vi "Instrument_Setting.vi"(8 "错误输入（无错误）":errorcluster, 9 "id":string[](array[string]), 10 "Get_USB_Resouce":string[](array[string]), 11 "Address Cluster":T2={"SPU"=refnum, "MPM"=[], "Port_Count"=0.0, "MPM_Count"=0.0, "SPU_Resource"=[], "USB_Resource"=[], "MPM_Communicater"="", "MPM_Count"=0.0, "MPM_Address"=[], "MPM_Portnumber"=[], "SPU_DeviveID"="", "MPM_communcation_method"=[], "TSL_sweepstartwave"=0.0, "TSL_sweepstopwave"=0.0, "TSL_Address"="", "TSL_Communicater"="", "TSL"=refnum, "tsl_communcation_method"=3, "TSL_Portnumber"=0.0, "PCU"=refnum, "PCU_Communicater"="", "PCU_Address"="", "PCU_Portnumber"=0.0, "PCU_useing_internal_DAQ"=FALSE, "PCU_communcation_method"=0} {"PCU_communcation_method" items=["GPIB", "C232C", "TCPIP", "USB"]; "tsl_communcation_method" items=["GPIB", "C232C", "TCPIP", "USB"]; "MPM_communcation_method" items=["GPIB", "C232C", "TCPIP", "USB"]}) -> (0 "错误输出":errorcluster, 2 "PowerMonitorType":enum16{"DAQ", "MPM_220", "TSL_LOGG"}(ring), 3 "Address Cluster out":T2={"SPU"=refnum, "MPM"=[], "Port_Count"=0.0, "MPM_Count"=0.0, "SPU_Resource"=[], "USB_Resource"=[], "MPM_Communicater"="", "MPM_Count"=0.0, "MPM_Address"=[], "MPM_Portnumber"=[], "SPU_DeviveID"="", "MPM_communcation_method"=[], "TSL_sweepstartwave"=0.0, "TSL_sweepstopwave"=0.0, "TSL_Address"="", "TSL_Communicater"="", "TSL"=refnum, "tsl_communcation_method"=3, "TSL_Portnumber"=0.0, "PCU"=refnum, "PCU_Communicater"="", "PCU_Address"="", "PCU_Portnumber"=0.0, "PCU_useing_internal_DAQ"=FALSE, "PCU_communcation_method"=0} {"PCU_communcation_method" items=["GPIB", "C232C", "TCPIP", "USB"]; "tsl_communcation_method" items=["GPIB", "C232C", "TCPIP", "USB"]; "MPM_communcation_method" items=["GPIB", "C232C", "TCPIP", "USB"]})   [LabVIEW 2017]
doc: "Setting Form"
uses:
  CTL/Address Cluster.ctl
  D:/test/PDLSTS/LV_PDL LvVer17.0/LV_PDL_x64/DLL/InstrumentDLL.dll
  DLL/InstrumentDLL.dll
  Share/Product_PCU.vi
  Share/MPM_PowerMonitorType.vi
panel:
  out "Enable220Flag":bool
  in  "Preformence":enum32{"High-Spec", "Standard"}(radio) caption="Preformance"
  in  "Product_MPM":enum32{"MPM-210/210H", "MPM-220"}(radio) caption="Product"
  in  "txtpcu_ipadd":string caption="IP Address"
  in  "txtpcu_lanport":i32=5000 caption="LAN Port"
  in  "txtpcu_gpibadd":i32=1 caption="GPIB Address"
  in  "cmbpcu_usbresource":u16(ring) caption="Usb resouce"
  in  "Communication_PCU":T1(radio) caption="Communication"
  in  "Product_PCU":enum32{"rdopcu100", "rdopcu110"}(radio) caption="Product"
  out "Boolean":bool=TRUE
  in  "Port_Count":i32
  in  "btnconnect":bool
  in  "cmbSPU_dev":u16(ring) caption="SPU" items=["Dev3"]
  in  "IP Address_MPM 2":string caption="IP Address"
  in  "LAN Port_MPM 2":dbl caption="LAN Port"
  in  "GPIB Address_MPM 2":i32 caption="GPIB Address"
  in  "chkmulti_dev":bool
  in  "IP Address_MPM":string caption="IP Address"
  in  "LAN Port_MPM":dbl=5000.0 caption="LAN Port"
  in  "GPIB Address_MPM":i32=14 caption="GPIB Address"
  in  "Communication_MPM":enum32{"rdiGPIB_MPM", "rdiLAN_MPM"}(radio) caption="Communication"
  in  "IP Address_TSL1":string caption="IP Address"
  in  "LAN Port_TSL1":i32 caption="LAN Port"
  in  "GPIB Address_TSL1":i32=1 caption="GPIB Address"
  in  "Usb resouce_TSL1":u16(ring) caption="Usb resouce"
  in  "Communication_TSL":T3(radio) caption="Communication"
  in  "Product_TSL":enum32{"rdo550_TSL", "rdo570_TSL"}(radio) caption="Product"
  # "TSL"
  # "MPM"
  # "Device2"
  # "Device1"
  # "PCU"
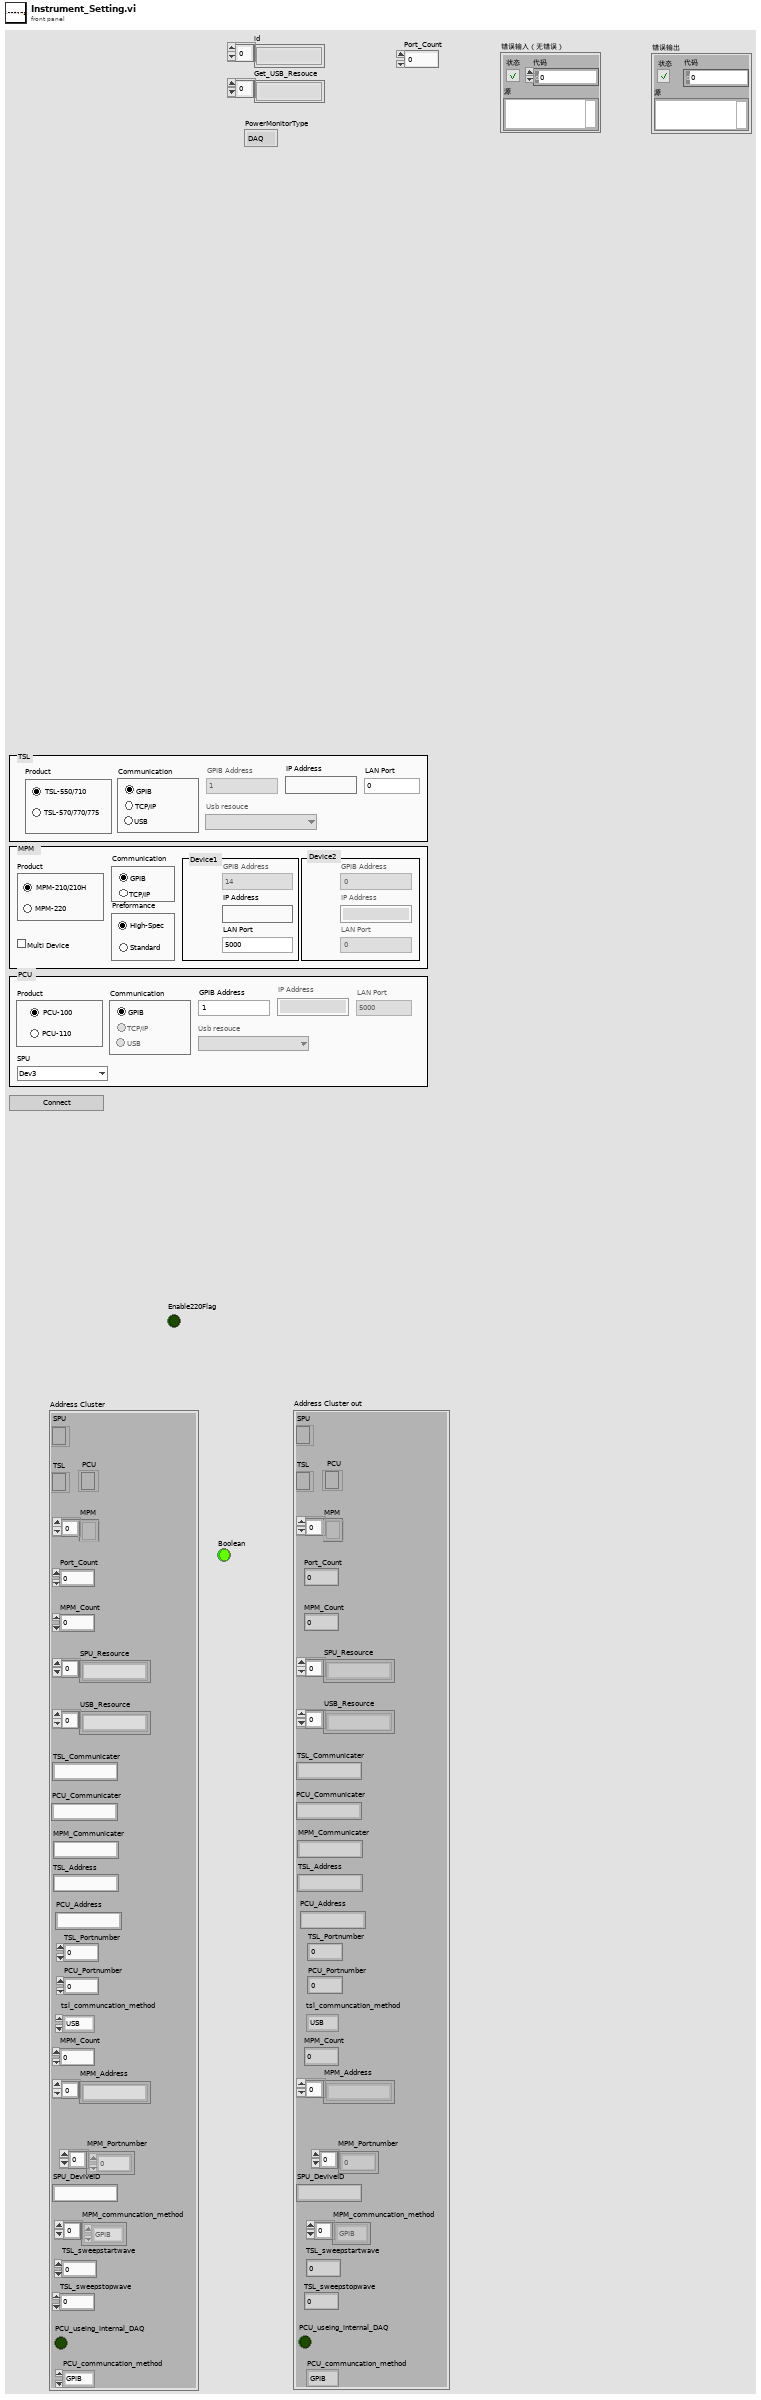
[diagram p1: front panel]
types:
  T1 = enum32{"rdopcu_gpib", "rdopcu_lan", "rdopcu_usb"}
  T2 = typedef "Address Cluster.ctl" = cluster{"SPU":refnum<k24>, "MPM":refnum<k24>[], "Port_Count":dbl, "MPM_Count":dbl, "SPU_Resource":string[], "USB_Resource":string[], "MPM_Communicater":string, "MPM_Count":dbl, "MPM_Address":string[], "MPM_Portnumber":dbl[], "SPU_DeviveID":string, "MPM_communcation_method":i32[], "TSL_sweepstartwave":dbl, "TSL_sweepstopwave":dbl, "TSL_Address":string, "TSL_Communicater":string, "TSL":refnum<k24>, "tsl_communcation_method":i32, "TSL_Portnumber":dbl, "PCU":refnum<k24>, "PCU_Communicater":string, "PCU_Address":string, "PCU_Portnumber":dbl, "PCU_useing_internal_DAQ":bool, "PCU_communcation_method":i32}
  T3 = enum32{"rdiGPIB_TSL", "rdiLAN_TSL", "rdiUSB_TSL"}
  T4 = enum8{"Enabled", "Disabled", "Disabled and Grayed Out"}
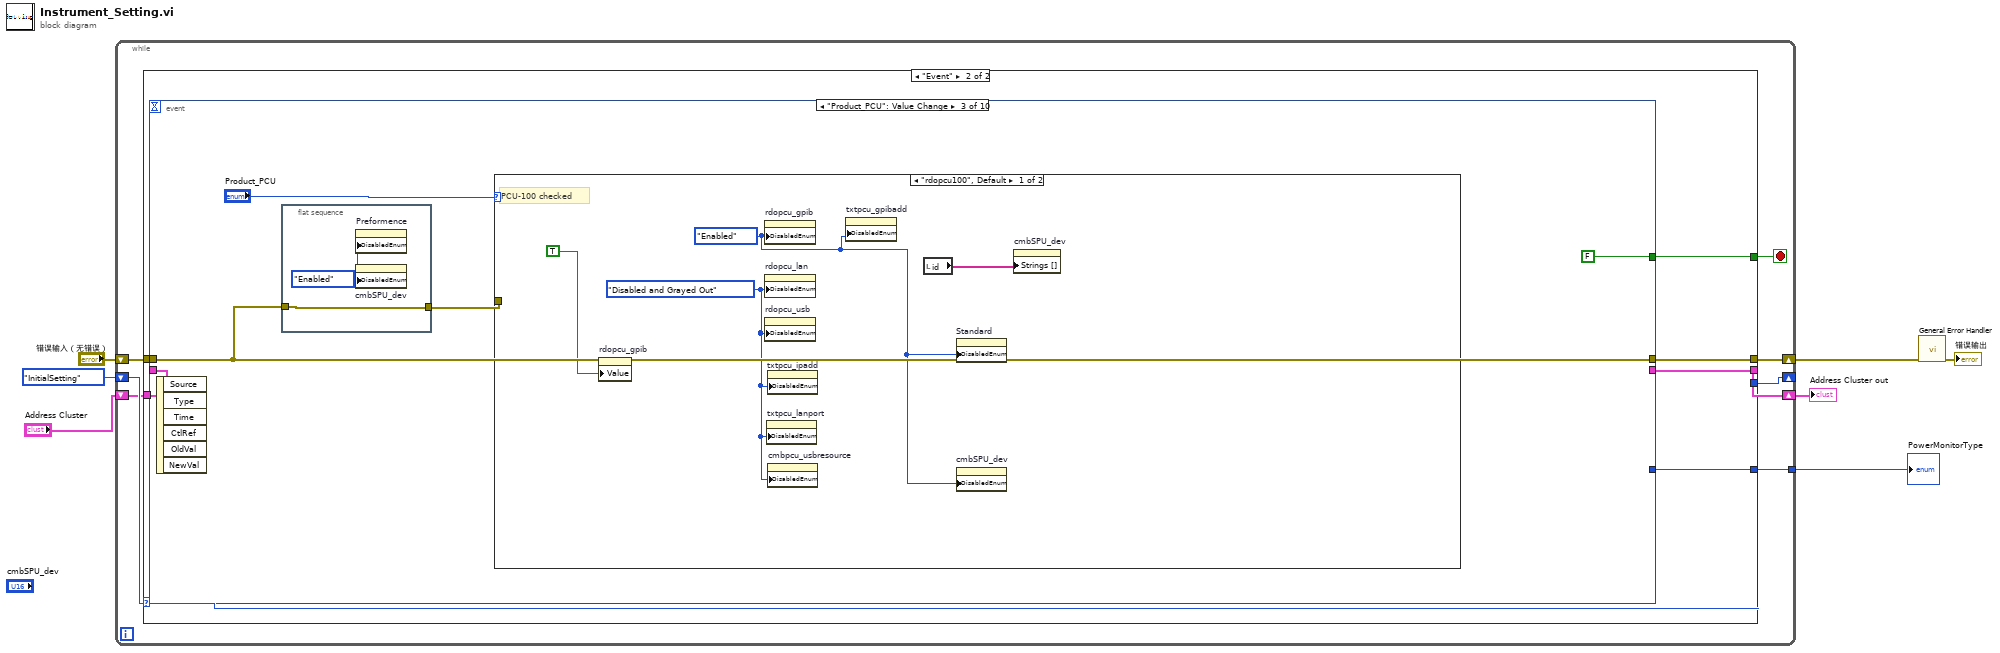
[diagram p0: block diagram]
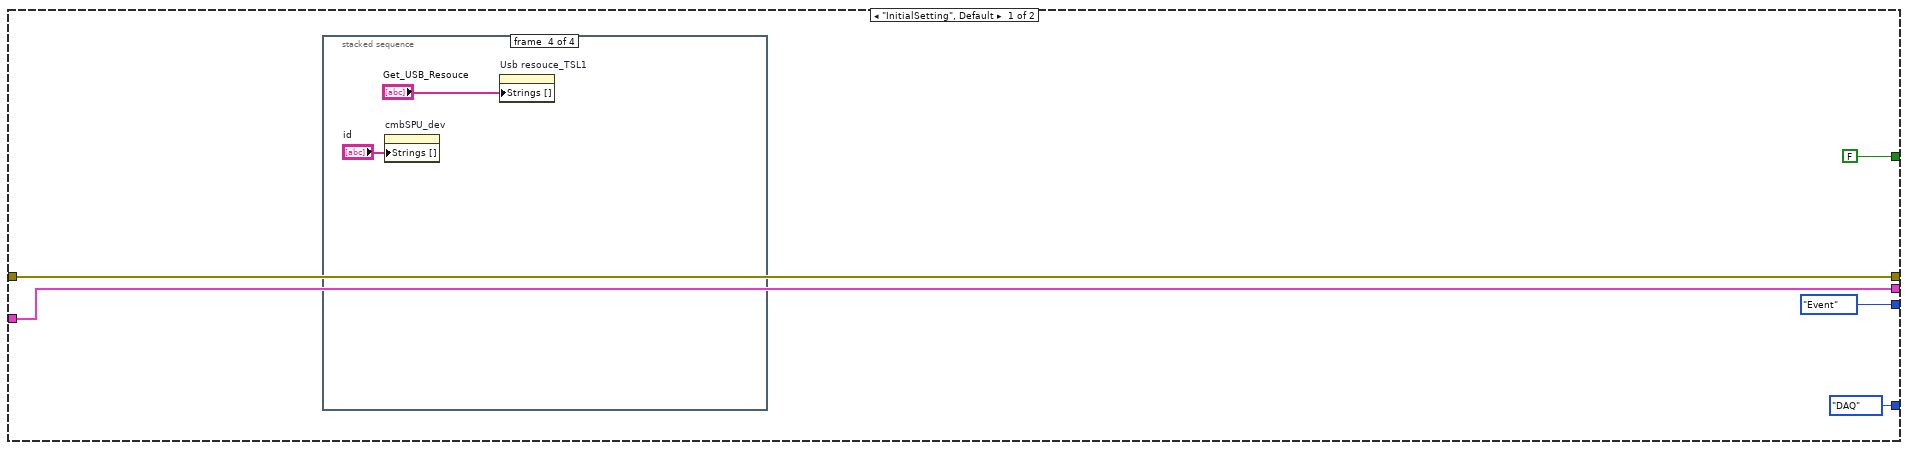
[diagram p2: hidden frame]
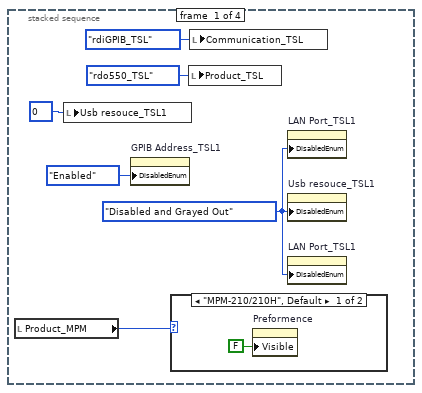
[diagram p3: hidden frame]
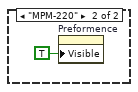
[diagram p4: hidden frame]
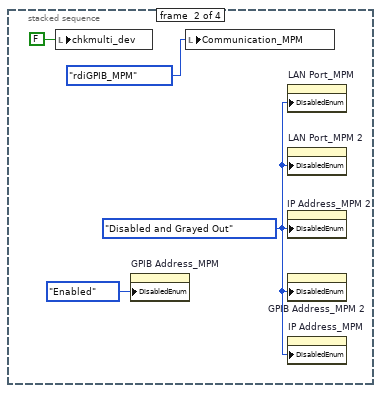
[diagram p5: hidden frame]
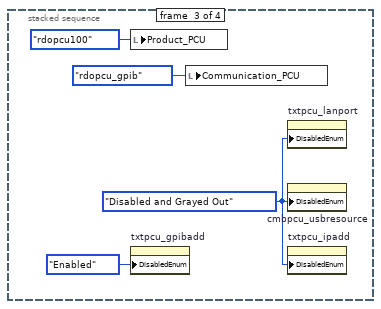
[diagram p6: hidden frame]
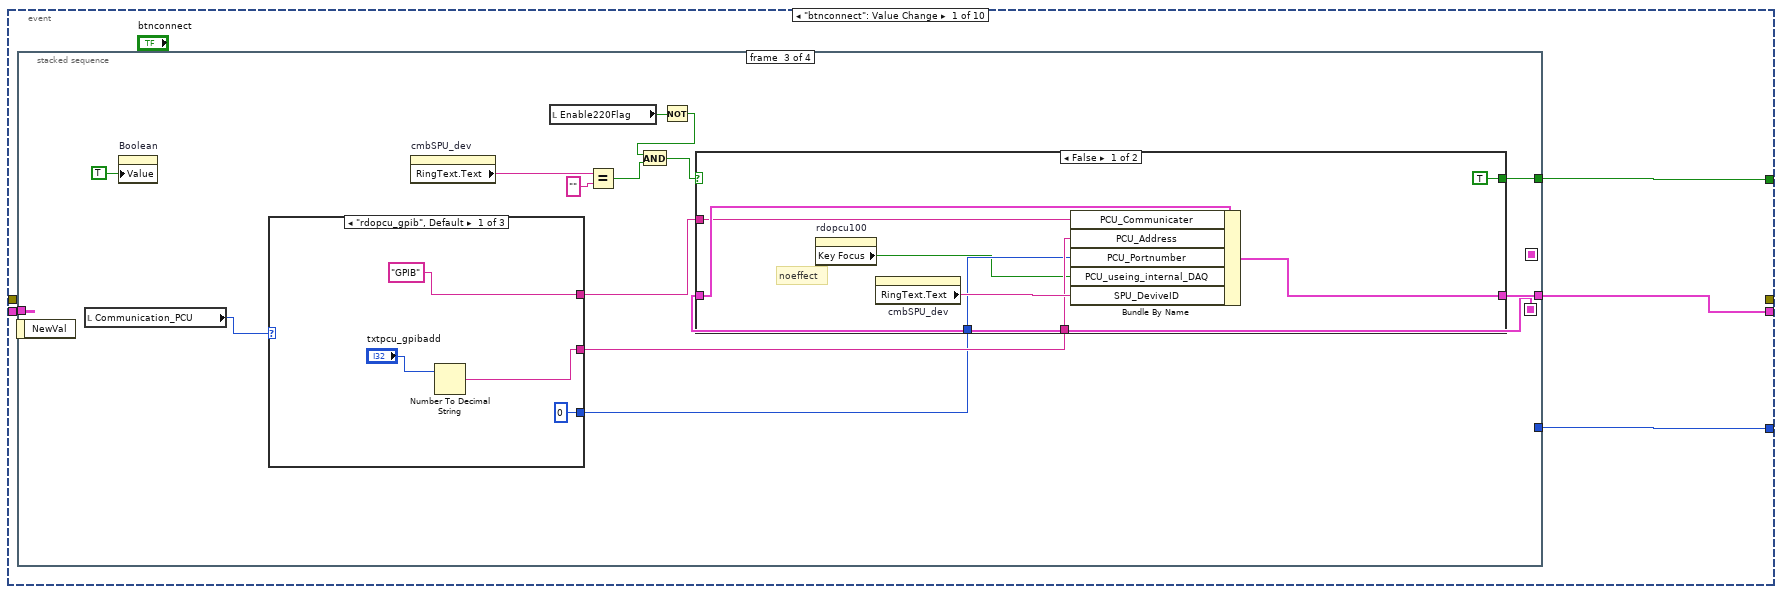
[diagram p7: hidden frame]
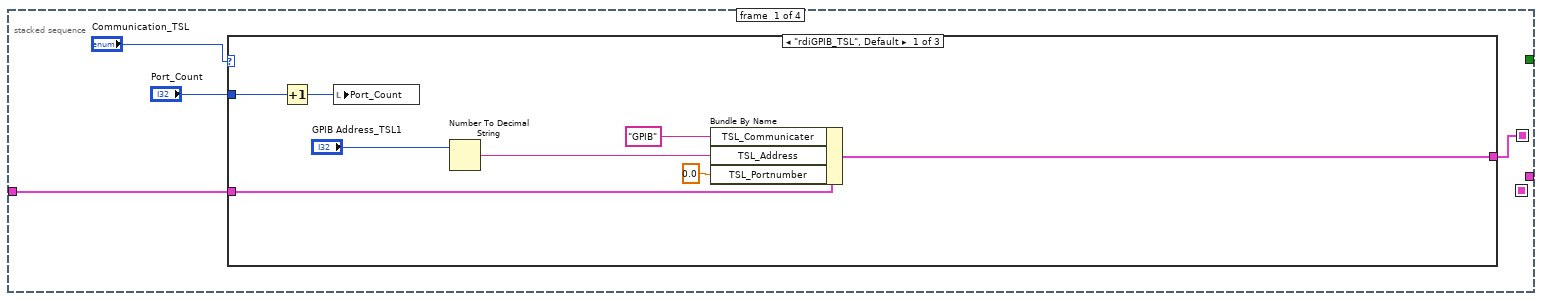
[diagram p8: hidden frame]
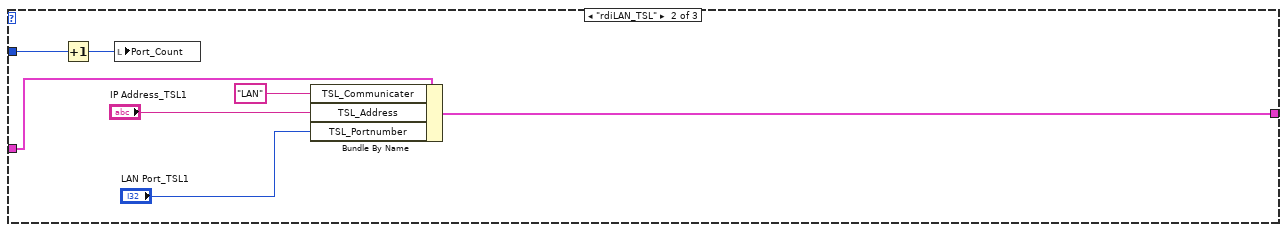
[diagram p9: hidden frame]
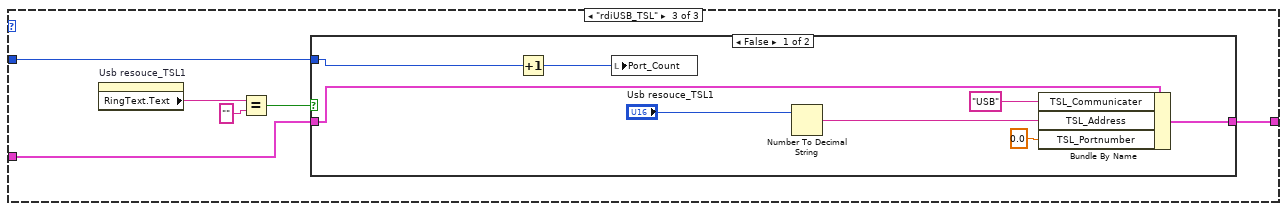
[diagram p10: hidden frame]
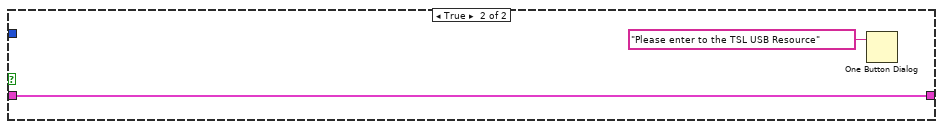
[diagram p11: hidden frame]
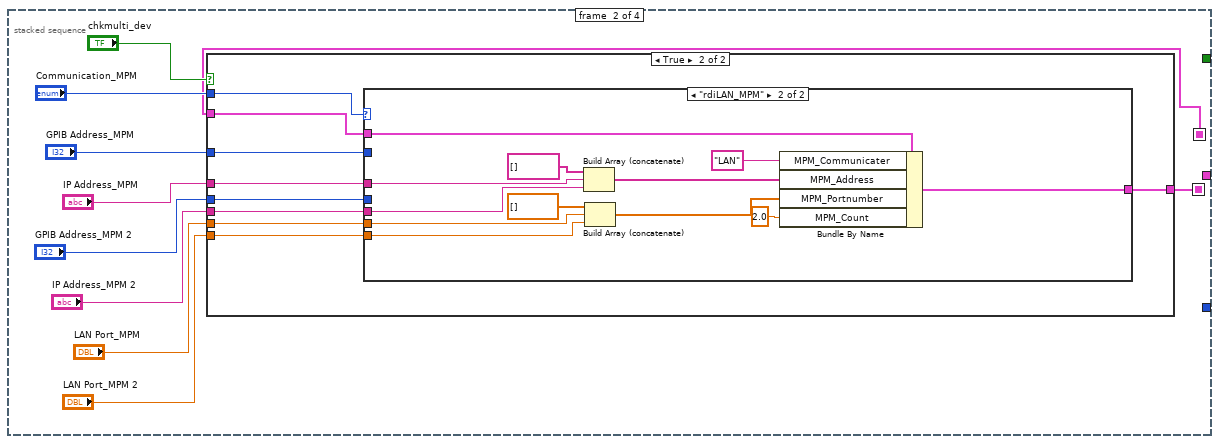
[diagram p12: hidden frame]
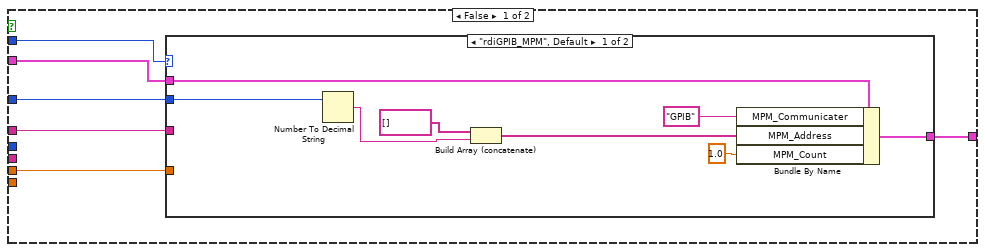
[diagram p13: hidden frame]
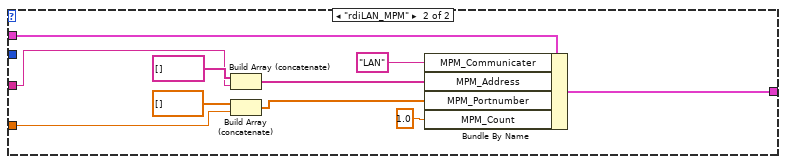
[diagram p14: hidden frame]
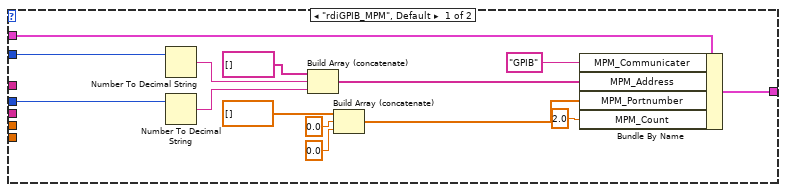
[diagram p15: hidden frame]
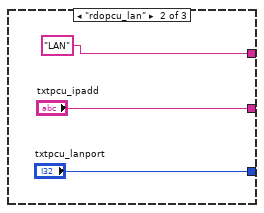
[diagram p16: hidden frame]
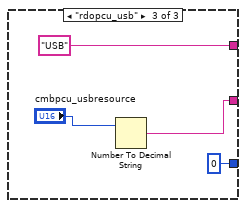
[diagram p17: hidden frame]
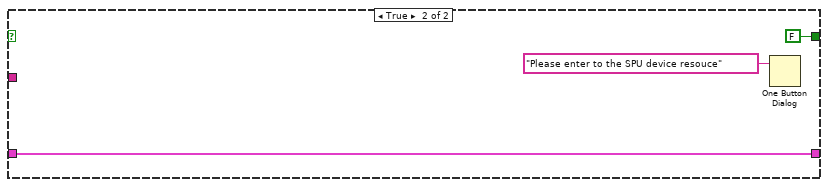
[diagram p18: hidden frame]
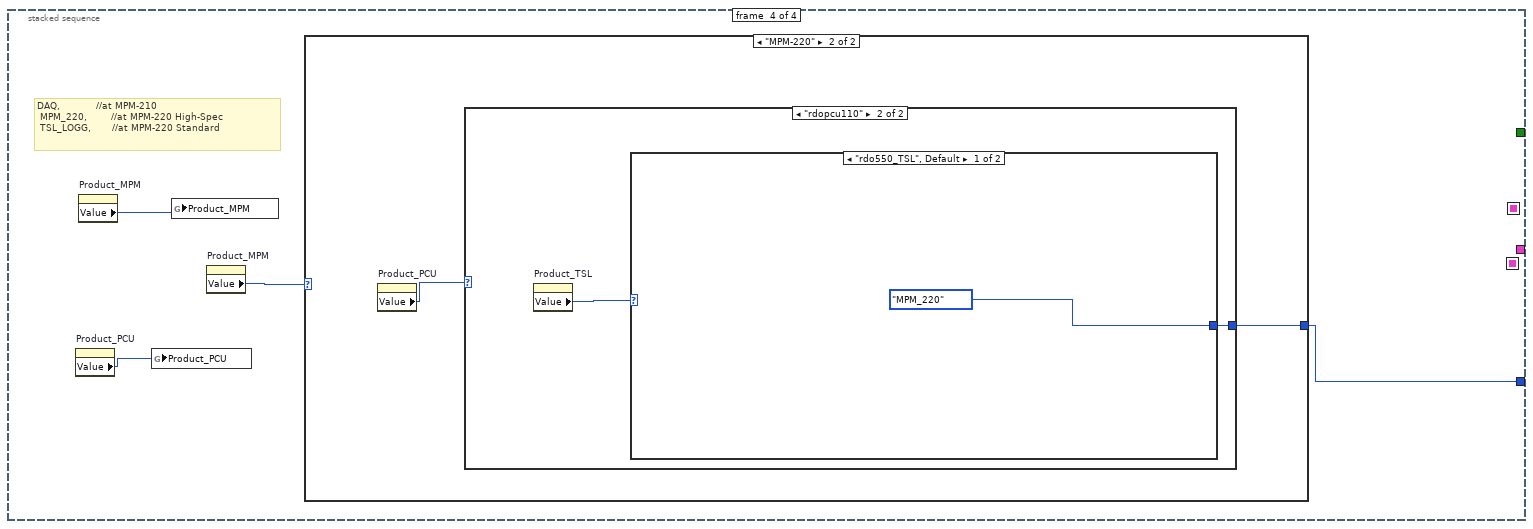
[diagram p19: hidden frame]
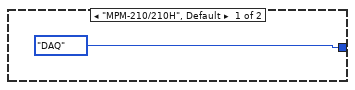
[diagram p20: hidden frame]
diagram:
  n1 = while {
    shift-right: [w14] -> w5
    shift-left: "错误输入（无错误）" -> [w15]
    shift-right: [w12] -> _
    shift-left: enum16{"InitialSetting", "Event", "Set", "Exit"}."InitialSetting" -> [w13]
    shift-right: [w10] -> w2
    shift-left: "Address Cluster" -> [w11]
    tunnel: [w8] -> w1
    stop <- w9 stop-if-true
    n2 = case shown="\"Event\"" w13 {
      selector: w13 -> [_ w41]
      tunnel: w15 -> [w17 w45]
      tunnel: [w17 w44] -> w14
      tunnel: [FALSE ("status") w40] -> w9
      tunnel: [enum16{"InitialSetting", "Event", "Set", "Exit"}."Event" w41] -> w12
      tunnel: w11 -> [w18 w43]
      tunnel: [w18 w42] -> w10
      tunnel: [enum16{"DAQ", "MPM_220", "TSL_LOGG"}."DAQ" ("f") w39] -> w8
      frame "InitialSetting", Default {
        n3 = stacked-sequence {
          frame #0 {
            w25 = T4."Disabled and Grayed Out" ("禁用")
            w26 = u16 0 items=[""] ("Usb resouce_TSL1")
            n4 = local read "Product_MPM"() -> (w21:enum32{"MPM-210/210H", "MPM-220"})
            n5 = local write "Usb resouce_TSL1"(w26) -> ()
            n6 = property on="GPIB Address_TSL1" class="DigNum (strict)"("DisabledEnum"=T4."Enabled" ("禁用")) -> ()  [unwired: 2 in, 2 out]
            n7 = case shown="\"MPM-210/210H\", Default" w21 {
              frame "MPM-210/210H", Default {
                n8 = property on="Preformence" class="RadioBtnsControl (strict)"("Visible"=FALSE) -> ()  [unwired: 2 in, 2 out]
              }
              frame "MPM-220" {
                n9 = property on="Preformence" class="RadioBtnsControl (strict)"("Visible"=TRUE) -> ()  [unwired: 2 in, 2 out]
              }
            }
            n10 = local write "Product_TSL"(enum32{"rdo550_TSL", "rdo570_TSL"}."rdo550_TSL" ("Product_TSL")) -> ()
            n11 = local write "Communication_TSL"(T3."rdiGPIB_TSL" ("Communication_TSL")) -> ()
            n12 = property on="LAN Port_TSL1" class="DigNum (strict)"("DisabledEnum"=w25) -> ()  [unwired: 2 in, 2 out]
            n13 = property on="Usb resouce_TSL1" class="Ring (strict)"("DisabledEnum"=w25) -> ()  [unwired: 2 in, 2 out]
            n14 = property on="LAN Port_TSL1" class="DigNum (strict)"("DisabledEnum"=w25) -> ()  [unwired: 2 in, 2 out]
          }
          frame #1 {
            w29 = T4."Disabled and Grayed Out" ("禁用")
            n15 = local write "chkmulti_dev"(FALSE ("chkmulti_dev")) -> ()
            n16 = property on="GPIB Address_MPM" class="DigNum (strict)"("DisabledEnum"=T4."Enabled" ("禁用")) -> ()  [unwired: 2 in, 2 out]
            n17 = local write "Communication_MPM"(enum32{"rdiGPIB_MPM", "rdiLAN_MPM"}."rdiGPIB_MPM" ("Communication_MPM")) -> ()
            n18 = property on="LAN Port_MPM" class="DigNum (strict)"("DisabledEnum"=w29) -> ()  [unwired: 2 in, 2 out]
            n19 = property on="LAN Port_MPM 2" class="DigNum (strict)"("DisabledEnum"=w29) -> ()  [unwired: 2 in, 2 out]
            n20 = property on="IP Address_MPM 2" class="Str"("DisabledEnum"=w29) -> ()  [unwired: 2 in, 2 out]
            n21 = property on="GPIB Address_MPM 2" class="DigNum (strict)"("DisabledEnum"=w29) -> ()  [unwired: 2 in, 2 out]
            n22 = property on="IP Address_MPM" class="Str"("DisabledEnum"=w29) -> ()  [unwired: 2 in, 2 out]
          }
          frame #2 {
            w33 = T4."Disabled and Grayed Out" ("禁用")
            n23 = local write "Product_PCU"(enum32{"rdopcu100", "rdopcu110"}."rdopcu100" ("Product_PCU")) -> ()
            n24 = property on="txtpcu_gpibadd" class="DigNum (strict)"("DisabledEnum"=T4."Enabled" ("禁用")) -> ()  [unwired: 2 in, 2 out]
            n25 = local write "Communication_PCU"(T1."rdopcu_gpib" ("Communication_PCU")) -> ()
            n26 = property on="txtpcu_lanport" class="DigNum (strict)"("DisabledEnum"=w33) -> ()  [unwired: 2 in, 2 out]
            n27 = property on="cmbpcu_usbresource" class="Ring (strict)"("DisabledEnum"=w33) -> ()  [unwired: 2 in, 2 out]
            n28 = property on="txtpcu_ipadd" class="Str"("DisabledEnum"=w33) -> ()  [unwired: 2 in, 2 out]
          }
          frame #3 {
            n29 = property on="cmbSPU_dev" class="Ring (strict)"("Strings []"="id") -> ()  [unwired: 2 in, 2 out]
            n30 = property on="Usb resouce_TSL1" class="Ring (strict)"("Strings []"="Get_USB_Resouce") -> ()  [unwired: 2 in, 2 out]
          }
        }
      }
      frame "Event" {
        n31 = event shown="[2] \"Product_PCU\": Value Change" {
          selector: _ -> [_ _ _ _ _ _ _ _ _ _]
          dyn-events: _ -> [_ _ _ _ _ _ _ _ _ _]
          timeout: _ -> [_ _ _ _ _ _ _ _ _ _]
          tunnel: w45 -> [_ w212 w231 w256 w273 w274 _ w290 w299 _]
          tunnel: [_ w212 w231 w256 w273 w274 _ w290 w299 _] -> w44
          tunnel: w43 -> [w49 _ _ _ _ _ _ _ _ w314]
          tunnel: [w48 _ _ _ _ _ _ _ _ w314] -> w42
          tunnel: [w47 FALSE ("y") FALSE ("y") _ _ FALSE ("y") _ FALSE ("y") FALSE ("y") TRUE ("y")] -> w40
          tunnel: [w46 _ _ _ _ _ _ _ _ _] -> w39
          event "btnconnect": Value Change {
            n32 = event-data() -> ()  [unwired: 1 in, 1 out]
            n33 = stacked-sequence {
              seq-local: [w52 _ _ _] -> [_ w85 _ _]
              seq-local: [_ w86 _ _] -> [_ _ w163 _]
              tunnel: w49 -> [w53 _ _ _]
              tunnel: [_ _ w165 _] -> w48
              tunnel: [_ _ w164 _] -> w47
              tunnel: [_ _ _ w192] -> w46
              frame #0 {
                n34 = case shown="\"rdiGPIB_TSL\", Default" "Communication_TSL" {
                  tunnel: "Port_Count" -> [w57 w66 w71]
                  tunnel: w53 -> [w60 w68 w70]
                  tunnel: [w59 w67 w69] -> w52
                  frame "rdiGPIB_TSL", Default {
                    n35 = Increment(x=w57) -> (x+1=w58:i32)
                    n36 = local write "Port_Count"(w58) -> ()
                    n37 = Number To Decimal String(number="GPIB Address_TSL1") -> (decimal integer string=w55:string)  [unwired: 1 in]
                    n38 = Bundle By Name(cluster=w60, "TSL_Communicater"="GPIB" ("新元素/子数组"), "TSL_Address"=w55, "TSL_Portnumber"=0.0 ("新元素/子数组")) -> (w59:T2)
                  }
                  frame "rdiLAN_TSL" {
                    n39 = Increment(x=w66) -> (x+1=w65:i32)
                    n40 = local write "Port_Count"(w65) -> ()
                    n41 = Bundle By Name(cluster=w68, "TSL_Communicater"="LAN" ("新元素/子数组"), "TSL_Address"="IP Address_TSL1", "TSL_Portnumber"="LAN Port_TSL1") -> (w67:T2)
                  }
                  frame "rdiUSB_TSL" {
                    n42 = property on="Usb resouce_TSL1" class="Ring (strict)"() -> ("RingText.Text"=w74:string)  [unwired: 2 in, 2 out]
                    n43 = Equal?(x=w74, y="") -> (x = y?=w72:bool)
                    n44 = case shown="False" w72 {
                      tunnel: w71 -> [w78 _]
                      tunnel: w70 -> [w81 w83]
                      tunnel: [w80 w83] -> w69
                      frame False {
                        n45 = Increment(x=w78) -> (x+1=w79:i32)
                        n46 = local write "Port_Count"(w79) -> ()
                        n47 = Number To Decimal String(number="Usb resouce_TSL1") -> (decimal integer string=w76:string)  [unwired: 1 in]
                        n48 = Bundle By Name(cluster=w81, "TSL_Communicater"="USB" ("新元素/子数组"), "TSL_Address"=w76, "TSL_Portnumber"=0.0 ("新元素/子数组")) -> (w80:T2)
                      }
                      frame True {
                        n49 = One Button Dialog(message="Please enter to the TSL USB Resource" ("消息")) -> ()  [unwired: 1 in, 1 out]
                      }
                    }
                  }
                }
              }
              frame #1 {
                n50 = case shown="True" "chkmulti_dev" {
                  tunnel: w85 -> [w96 w127]
                  tunnel: "Communication_MPM" -> [w100 w126]
                  tunnel: [w97 w125] -> w86
                  tunnel: "GPIB Address_MPM 2" -> [_ w124]
                  tunnel: "GPIB Address_MPM" -> [w95 w123]
                  tunnel: "LAN Port_MPM 2" -> [_ w122]
                  tunnel: "LAN Port_MPM" -> [w99 w121]
                  tunnel: "IP Address_MPM 2" -> [_ w120]
                  tunnel: "IP Address_MPM" -> [w98 w119]
                  frame False {
                    n51 = case shown="\"rdiGPIB_MPM\", Default" w100 {
                      tunnel: w99 -> [_ w115]
                      tunnel: w98 -> [_ w112]
                      tunnel: [w105 w110] -> w97
                      tunnel: w96 -> [w106 w109]
                      tunnel: w95 -> [w102 _]
                      frame "rdiGPIB_MPM", Default {
                        n52 = Number To Decimal String(number=w102) -> (decimal integer string=w103:string)  [unwired: 1 in]
                        n53 = Build Array (concatenate)(string[] [] ("MPM_Address"), w103) -> (w101:string[])
                        n54 = Bundle By Name(cluster=w106, "MPM_Communicater"="GPIB", "MPM_Address"=w101, "MPM_Count"=1.0) -> (w105:T2)
                      }
                      frame "rdiLAN_MPM" {
                        n55 = Build Array (concatenate)(string[] [] ("MPM_Address"), w112) -> (w111:string[])
                        n56 = Build Array (concatenate)(dbl[] [] ("MPM_Portnumber"), w115) -> (w114:dbl[])
                        n57 = Bundle By Name(cluster=w109, "MPM_Communicater"="LAN", "MPM_Address"=w111, "MPM_Portnumber"=w114, "MPM_Count"=1.0) -> (w110:T2)
                      }
                    }
                  }
                  frame True {
                    n58 = case shown="\"rdiLAN_MPM\"" w126 {
                      tunnel: w127 -> [w135 w153]
                      tunnel: [w130 w142] -> w125
                      tunnel: w124 -> [w129 _]
                      tunnel: w123 -> [w128 _]
                      tunnel: w122 -> [_ w146]
                      tunnel: w121 -> [_ w145]
                      tunnel: w120 -> [_ w144]
                      tunnel: w119 -> [_ w143]
                      frame "rdiGPIB_MPM", Default {
                        n59 = Number To Decimal String(number=w128) -> (decimal integer string=w138:string)  [unwired: 1 in]
                        n60 = Number To Decimal String(number=w129) -> (decimal integer string=w137:string)  [unwired: 1 in]
                        n61 = Build Array (concatenate)(string[] [] ("MPM_Address"), w138, w137) -> (w136:string[])
                        n62 = Build Array (concatenate)(dbl[] [] ("MPM_Portnumber"), 0.0 ("新元素/子数组"), 0.0 ("新元素/子数组")) -> (w131:dbl[])
                        n63 = Bundle By Name(cluster=w135, "MPM_Communicater"="GPIB", "MPM_Address"=w136, "MPM_Portnumber"=w131, "MPM_Count"=2.0) -> (w130:T2)
                      }
                      frame "rdiLAN_MPM" {
                        n64 = Build Array (concatenate)(string[] [] ("MPM_Address"), w143, w144) -> (w149:string[])
                        n65 = Build Array (concatenate)(dbl[] [] ("MPM_Portnumber"), w145, w146) -> (w147:dbl[])
                        n66 = Bundle By Name(cluster=w153, "MPM_Communicater"="LAN", "MPM_Address"=w149, "MPM_Portnumber"=w147, "MPM_Count"=2.0) -> (w142:T2)
                      }
                    }
                  }
                }
              }
              frame #2 {
                n67 = local read "Communication_PCU"() -> (w161:T1)
                n68 = property on="Boolean" class="Bool (strict)"("Value"=TRUE ("Boolean")) -> ()  [unwired: 2 in, 2 out]
                n69 = case shown="\"rdopcu_gpib\", Default" w161 {
                  tunnel: ["GPIB" "LAN" "USB"] -> w160
                  tunnel: [w169 "txtpcu_ipadd" w176] -> w159
                  tunnel: [0 ("txtpcu_lanport") "txtpcu_lanport" 0 ("txtpcu_lanport")] -> w158
                  frame "rdopcu_gpib", Default {
                    n70 = Number To Decimal String(number="txtpcu_gpibadd") -> (decimal integer string=w169:string)  [unwired: 1 in]
                  }
                  frame "rdopcu_lan" {
                  }
                  frame "rdopcu_usb" {
                    n71 = Number To Decimal String(number="cmbpcu_usbresource") -> (decimal integer string=w176:string)  [unwired: 1 in]
                  }
                }
                n72 = property on="cmbSPU_dev" class="Ring (strict)"() -> ("RingText.Text"=w167:string)  [unwired: 2 in, 2 out]
                n73 = local read "Enable220Flag"() -> (w155:bool)
                n74 = Equal?(x=w167, y="") -> (x = y?=w157:bool)
                n75 = Not(x=w155) -> (.not. x?=w154:bool)
                n76 = And(x=w154, y=w157) -> (x .and. y?=w156:bool)
                n77 = case shown="False" w156 {
                  tunnel: w163 -> [w186 w188]
                  tunnel: [w185 w188] -> w165
                  tunnel: [TRUE ("y") FALSE ("y")] -> w164
                  tunnel: w160 -> [w182 _]
                  tunnel: w159 -> [w181 _]
                  tunnel: w158 -> [w180 _]
                  frame False {
                    # "noeffect"
                    n78 = property on="rdopcu100" class="Bool (strict)"() -> ("Key Focus"=w179:bool)  [unwired: 2 in, 2 out]
                    n79 = property on="cmbSPU_dev" class="Ring (strict)"() -> ("RingText.Text"=w184:string)  [unwired: 2 in, 2 out]
                    n80 = Bundle By Name(cluster=w186, "PCU_Communicater"=w182, "PCU_Address"=w181, "PCU_Portnumber"=w180, "PCU_useing_internal_DAQ"=w179, "SPU_DeviveID"=w184) -> (w185:T2)
                  }
                  frame True {
                    n81 = One Button Dialog(message="Please enter to the SPU device resouce" ("消息")) -> ()  [unwired: 1 in, 1 out]
                  }
                }
              }
              frame #3 {
                # "DAQ,            //at MPM-210\n MPM_220,        //at MPM-220 High-Spec\n TSL_LOGG,       //at MPM-220 Standard"
                n82 = property on="Product_PCU" class="RadioBtnsControl (strict)"() -> ("Value"=w191:enum32{"rdopcu100", "rdopcu110"})  [unwired: 2 in, 2 out]
                n83 = property on="Product_MPM" class="RadioBtnsControl (strict)"() -> ("Value"=w190:enum32{"MPM-210/210H", "MPM-220"})  [unwired: 2 in, 2 out]
                n84 = global write "Product_PCU.vi" "Product_PCU"(w191) -> ()
                n85 = global write "MPM_PowerMonitorType.vi" "Product_MPM"(w190) -> ()
                n86 = property on="Product_MPM" class="RadioBtnsControl (strict)"() -> ("Value"=w193:enum32{"MPM-210/210H", "MPM-220"})  [unwired: 2 in, 2 out]
                n87 = case shown="\"MPM-220\"" w193 {
                  tunnel: [enum16{"DAQ", "MPM_220", "TSL_LOGG"}."DAQ" ("PowerMonitorType") w195] -> w192
                  frame "MPM-210/210H", Default {
                  }
                  frame "MPM-220" {
                    n88 = property on="Product_PCU" class="RadioBtnsControl (strict)"() -> ("Value"=w196:enum32{"rdopcu100", "rdopcu110"})  [unwired: 2 in, 2 out]
                    n89 = case shown="\"rdopcu110\"" w196 {
                      tunnel: [w197 w203] -> w195
                      frame "rdopcu100", Default {
                        n90 = property on="Preformence" class="RadioBtnsControl (strict)"() -> ("Value"=w202:enum32{"High-Spec", "Standard"})  [unwired: 2 in, 2 out]
                        n91 = Equal?(x=w202, y=enum32{"High-Spec", "Standard"}."High-Spec") -> (x = y?=w200:bool)
                        n92 = Select(t=enum16{"DAQ", "MPM_220", "TSL_LOGG"}."MPM_220" ("PowerMonitorType"), s=w200, f=enum16{"DAQ", "MPM_220", "TSL_LOGG"}."DAQ") -> (s? t:f=w197:enum16{"DAQ", "MPM_220", "TSL_LOGG"})
                      }
                      frame "rdopcu110" {
                        n93 = property on="Product_TSL" class="RadioBtnsControl (strict)"() -> ("Value"=w204:enum32{"rdo550_TSL", "rdo570_TSL"})  [unwired: 2 in, 2 out]
                        n94 = case shown="\"rdo550_TSL\", Default" w204 {
                          tunnel: [enum16{"DAQ", "MPM_220", "TSL_LOGG"}."MPM_220" ("PowerMonitorType") w206] -> w203
                          frame "rdo550_TSL", Default {
                          }
                          frame "rdo570_TSL" {
                            n95 = property on="Preformence" class="RadioBtnsControl (strict)"() -> ("Value"=w209:enum32{"High-Spec", "Standard"})  [unwired: 2 in, 2 out]
                            n96 = Equal?(x=w209, y=enum32{"High-Spec", "Standard"}."High-Spec") -> (x = y?=w207:bool)
                            n97 = Select(t=enum16{"DAQ", "MPM_220", "TSL_LOGG"}."MPM_220" ("PowerMonitorType"), s=w207, f=enum16{"DAQ", "MPM_220", "TSL_LOGG"}."TSL_LOGG") -> (s? t:f=w206:enum16{"DAQ", "MPM_220", "TSL_LOGG"})
                          }
                        }
                      }
                    }
                  }
                }
              }
            }
          }
          event "Product_TSL": Value Change {
            n98 = event-data() -> ()  [unwired: 1 in, 1 out]
            n99 = flat-sequence {
              tunnel: [w216] -> w213
              tunnel: w212 -> [w216]
              frame #0 {
                n100 = property on="Preformence" class="RadioBtnsControl (strict)"("DisabledEnum"=T4."Enabled" ("Disabled")) -> ()  [unwired: 2 in, 2 out]
              }
            }
            n101 = case shown="\"rdo570_TSL\"" "Product_TSL" {
              tunnel: w213 -> [_ _]
              frame "rdo550_TSL", Default {
                w226 = T4."Disabled and Grayed Out" ("禁用")
                # "'TSL-550/710\n' There can control only GPIB"
                n102 = property on="rdiGPIB_TSL" class="Bool (strict)"("Value"=TRUE ("键选中")) -> ()  [unwired: 2 in, 2 out]
                n103 = property on="Product_MPM" class="RadioBtnsControl (strict)"() -> ("Value"=w224:enum32{"MPM-210/210H", "MPM-220"})  [unwired: 2 in, 2 out]
                n104 = property on="Product_PCU" class="RadioBtnsControl (strict)"() -> ("Value"=w223:enum32{"rdopcu100", "rdopcu110"})  [unwired: 2 in, 2 out]
                n105 = property on="rdiLAN_TSL" class="Bool (strict)"("DisabledEnum"=w226) -> ()  [unwired: 2 in, 2 out]
                n106 = property on="rdiUSB_TSL" class="Bool (strict)"("DisabledEnum"=w226) -> ()  [unwired: 2 in, 2 out]
                n107 = Equal?(x=w224, y=enum32{"MPM-210/210H", "MPM-220"}."MPM-220") -> (x = y?=w219:bool)
                n108 = Equal?(x=w223, y=enum32{"rdopcu100", "rdopcu110"}."rdopcu110") -> (x = y?=w218:bool)
                n109 = And(x=w219, y=w218) -> (x .and. y?=w220:bool)
                n110 = case shown="True" w220 {
                  frame False {
                  }
                  frame True {
                    n111 = property on="Preformence" class="RadioBtnsControl (strict)"("Value"=enum32{"High-Spec", "Standard"}."High-Spec" ("t")) -> ()  [unwired: 2 in, 2 out]
                    n112 = property on="Preformence" class="RadioBtnsControl (strict)"("DisabledEnum"=T4."Disabled and Grayed Out" ("t")) -> ()  [unwired: 2 in, 2 out]
                  }
                }
              }
              frame "rdo570_TSL" {
                w229 = T4."Enabled" ("禁用")
                # "TSL-570"
                n113 = property on="rdiLAN_TSL" class="Bool (strict)"("DisabledEnum"=w229) -> ()  [unwired: 2 in, 2 out]
                n114 = property on="rdiUSB_TSL" class="Bool (strict)"("DisabledEnum"=w229) -> ()  [unwired: 2 in, 2 out]
              }
            }
          }
          event "Product_PCU": Value Change {
            n115 = event-data() -> ()  [unwired: 1 in, 6 out]
            n116 = flat-sequence {
              tunnel: w231 -> [w235]
              tunnel: [w235] -> w230
              frame #0 {
                w234 = T4."Enabled" ("Disabled")
                n117 = property on="Preformence" class="RadioBtnsControl (strict)"("DisabledEnum"=w234) -> ()  [unwired: 2 in, 2 out]
                n118 = property on="cmbSPU_dev" class="Ring (strict)"("DisabledEnum"=w234) -> ()  [unwired: 2 in, 2 out]
              }
            }
            n119 = case shown="\"rdopcu100\", Default" "Product_PCU" {
              tunnel: w230 -> [_ _]
              frame "rdopcu100", Default {
                w237 = T4."Enabled" ("禁用")
                w239 = T4."Disabled and Grayed Out" ("禁用")
                # "PCU-100 checked"
                n120 = property on="rdopcu_gpib" class="Bool (strict)"("Value"=TRUE ("键选中")) -> ()  [unwired: 2 in, 2 out]
                n121 = property on="rdopcu_gpib" class="Bool (strict)"("DisabledEnum"=w237) -> ()  [unwired: 2 in, 2 out]
                n122 = property on="rdopcu_lan" class="Bool (strict)"("DisabledEnum"=w239) -> ()  [unwired: 2 in, 2 out]
                n123 = property on="rdopcu_usb" class="Bool (strict)"("DisabledEnum"=w239) -> ()  [unwired: 2 in, 2 out]
                n124 = property on="txtpcu_lanport" class="DigNum (strict)"("DisabledEnum"=w239) -> ()  [unwired: 2 in, 2 out]
                n125 = property on="txtpcu_ipadd" class="Str"("DisabledEnum"=w239) -> ()  [unwired: 2 in, 2 out]
                n126 = property on="cmbpcu_usbresource" class="Ring (strict)"("DisabledEnum"=w239) -> ()  [unwired: 2 in, 2 out]
                n127 = property on="txtpcu_gpibadd" class="DigNum (strict)"("DisabledEnum"=w237) -> ()  [unwired: 2 in, 2 out]
                n128 = local read "id"() -> (w236:string[])
                n129 = property on="Standard" class="Bool (strict)"("DisabledEnum"=w237) -> ()  [unwired: 2 in, 2 out]
                n130 = property on="cmbSPU_dev" class="Ring (strict)"("DisabledEnum"=w237) -> ()  [unwired: 2 in, 2 out]
                n131 = property on="cmbSPU_dev" class="Ring (strict)"("Strings []"=w236) -> ()  [unwired: 2 in, 2 out]
              }
              frame "rdopcu110" {
                w248 = T4."Enabled" ("禁用")
                w249 = T4."Disabled and Grayed Out" ("禁用")
                # "PCU-110 checked"
                n132 = property on="rdopcu_gpib" class="Bool (strict)"("Key Focus"=TRUE ("键选中")) -> ()  [unwired: 2 in, 2 out]
                n133 = property on="rdopcu_gpib" class="Bool (strict)"("DisabledEnum"=w248) -> ()  [unwired: 2 in, 2 out]
                n134 = property on="txtpcu_lanport" class="DigNum (strict)"("DisabledEnum"=w249) -> ()  [unwired: 2 in, 2 out]
                n135 = property on="txtpcu_ipadd" class="Str"("DisabledEnum"=w249) -> ()  [unwired: 2 in, 2 out]
                n136 = property on="cmbpcu_usbresource" class="Ring (strict)"("DisabledEnum"=w249) -> ()  [unwired: 2 in, 2 out]
                n137 = property on="txtpcu_gpibadd" class="DigNum (strict)"("DisabledEnum"=w248) -> ()  [unwired: 2 in, 2 out]
                n138 = property on="rdopcu_lan" class="Bool (strict)"("DisabledEnum"=w248) -> ()  [unwired: 2 in, 2 out]
                n139 = property on="rdopcu_usb" class="Bool (strict)"("DisabledEnum"=w248) -> ()  [unwired: 2 in, 2 out]
                n140 = property on="Product_MPM" class="RadioBtnsControl (strict)"() -> ("Value"=w246:enum32{"MPM-210/210H", "MPM-220"})  [unwired: 2 in, 2 out]
                n141 = property on="Product_TSL" class="RadioBtnsControl (strict)"() -> ("Value"=w243:enum32{"rdo550_TSL", "rdo570_TSL"})  [unwired: 2 in, 2 out]
                n142 = Equal?(x=w243, y=enum32{"rdo550_TSL", "rdo570_TSL"}."rdo550_TSL") -> (x = y?=w245:bool)
                n143 = Equal?(x=w246, y=enum32{"MPM-210/210H", "MPM-220"}."MPM-220") -> (x = y?=w242:bool)
                n144 = And(x=w242, y=w245) -> (x .and. y?=w241:bool)
                n145 = case shown="True" w242 {
                  frame False {
                  }
                  frame True {
                    n146 = property on="cmbSPU_dev" class="Ring (strict)"("RingText.Text"="" ("y")) -> ()  [unwired: 2 in, 2 out]
                    n147 = property on="cmbSPU_dev" class="Ring (strict)"("DisabledEnum"=T4."Disabled and Grayed Out" ("Disabled")) -> ()  [unwired: 2 in, 2 out]
                  }
                }
                n148 = case shown="True" w241 {
                  frame False {
                  }
                  frame True {
                    n149 = property on="Preformence" class="RadioBtnsControl (strict)"("Value"=enum32{"High-Spec", "Standard"}."High-Spec" ("t")) -> ()  [unwired: 2 in, 2 out]
                    n150 = property on="Preformence" class="RadioBtnsControl (strict)"("DisabledEnum"=T4."Disabled and Grayed Out" ("t")) -> ()  [unwired: 2 in, 2 out]
                  }
                }
              }
            }
          }
          event "Product_MPM": Value Change {
            # "tsl550 mpm220 pcu110"
            n151 = event-data() -> ()  [unwired: 1 in, 6 out]
            n152 = flat-sequence {
              tunnel: w256 -> [w272]
              tunnel: [w272] -> w254
              frame #0 {
                n153 = property on="Preformence" class="RadioBtnsControl (strict)"("DisabledEnum"=T4."Enabled" ("Disabled")) -> ()  [unwired: 2 in, 2 out]
              }
            }
            n154 = case shown="\"MPM-220\"" "Product_MPM" {
              tunnel: w254 -> [_ _]
              frame "MPM-210/210H", Default {
                w258 = FALSE ("Visible")
                n155 = property on="Preformence" class="RadioBtnsControl (strict)"("Visible"=w258) -> ()  [unwired: 2 in, 2 out]
                n156 = local write "Enable220Flag"(w258) -> ()
                n157 = property on="cmbSPU_dev" class="Ring (strict)"("DisabledEnum"=T4."Enabled" ("Disabled")) -> ()  [unwired: 2 in, 2 out]
              }
              frame "MPM-220" {
                w260 = TRUE ("Visible")
                n158 = property on="Preformence" class="RadioBtnsControl (strict)"("Visible"=w260) -> ()  [unwired: 2 in, 2 out]
                n159 = property on="Product_PCU" class="RadioBtnsControl (strict)"() -> ("Value"=w263:enum32{"rdopcu100", "rdopcu110"})  [unwired: 2 in, 2 out]
                n160 = property on="Product_TSL" class="RadioBtnsControl (strict)"() -> ("Value"=w265:enum32{"rdo550_TSL", "rdo570_TSL"})  [unwired: 2 in, 2 out]
                n161 = Equal?(x=w263, y=enum32{"rdopcu100", "rdopcu110"}."rdopcu110") -> (x = y?=w261:bool)
                n162 = Equal?(x=w265, y=enum32{"rdo550_TSL", "rdo570_TSL"}."rdo550_TSL" ("Product_TSL")) -> (x = y?=w266:bool)
                n163 = And(x=w261, y=w266) -> (x .and. y?=w264:bool)
                n164 = case shown="True" w264 {
                  frame False {
                  }
                  frame True {
                    n165 = property on="Preformence" class="RadioBtnsControl (strict)"("Value"=enum32{"High-Spec", "Standard"}."High-Spec" ("t")) -> ()  [unwired: 2 in, 2 out]
                    n166 = property on="Preformence" class="RadioBtnsControl (strict)"("DisabledEnum"=T4."Disabled and Grayed Out" ("t")) -> ()  [unwired: 2 in, 2 out]
                  }
                }
                n167 = case shown="True" w261 {
                  frame False {
                  }
                  frame True {
                    n168 = property on="cmbSPU_dev" class="Ring (strict)"("RingText.Text"="" ("y")) -> ()  [unwired: 2 in, 2 out]
                    n169 = property on="cmbSPU_dev" class="Ring (strict)"("DisabledEnum"=T4."Disabled and Grayed Out" ("Disabled")) -> ()  [unwired: 2 in, 2 out]
                  }
                }
                "Enable220Flag" <- w260
              }
            }
          }
          event "Preformence": Value Change {
            n170 = event-data() -> ()  [unwired: 1 in, 6 out]
          }
          event "Communication_TSL": Value Change {
            n171 = event-data() -> ()  [unwired: 1 in, 1 out]
            n172 = local read "Communication_TSL"() -> (w276:T3)
            n173 = case shown="\"rdiGPIB_TSL\", Default" w276 {
              frame "rdiLAN_TSL" {
                w277 = T4."Enabled" ("禁用")
                w278 = T4."Disabled and Grayed Out" ("禁用")
                # "TSL Control TCP/IP"
                n174 = property on="IP Address_TSL1" class="Str"("DisabledEnum"=w277) -> ()  [unwired: 2 in, 2 out]
                n175 = property on="LAN Port_TSL1" class="DigNum (strict)"("DisabledEnum"=w277) -> ()  [unwired: 2 in, 2 out]
                n176 = property on="Usb resouce_TSL1" class="Ring (strict)"("DisabledEnum"=w278) -> ()  [unwired: 2 in, 2 out]
                n177 = property on="GPIB Address_TSL1" class="DigNum (strict)"("DisabledEnum"=w278) -> ()  [unwired: 2 in, 2 out]
              }
              frame "rdiGPIB_TSL", Default {
                w279 = T4."Disabled and Grayed Out" ("禁用")
                # "TSL Control GPIB"
                n178 = property on="GPIB Address_TSL1" class="DigNum (strict)"("DisabledEnum"=T4."Enabled" ("禁用")) -> ()  [unwired: 2 in, 2 out]
                n179 = property on="Usb resouce_TSL1" class="Ring (strict)"("DisabledEnum"=w279) -> ()  [unwired: 2 in, 2 out]
                n180 = property on="LAN Port_TSL1" class="DigNum (strict)"("DisabledEnum"=w279) -> ()  [unwired: 2 in, 2 out]
                n181 = property on="IP Address_TSL1" class="Str"("DisabledEnum"=w279) -> ()  [unwired: 2 in, 2 out]
              }
              frame "rdiUSB_TSL" {
                w281 = T4."Disabled and Grayed Out" ("禁用")
                # "TSL Control USB"
                n182 = property on="Usb resouce_TSL1" class="Ring (strict)"("DisabledEnum"=T4."Enabled" ("禁用")) -> ()  [unwired: 2 in, 2 out]
                n183 = property on="GPIB Address_TSL1" class="DigNum (strict)"("DisabledEnum"=w281) -> ()  [unwired: 2 in, 2 out]
                n184 = property on="LAN Port_TSL1" class="DigNum (strict)"("DisabledEnum"=w281) -> ()  [unwired: 2 in, 2 out]
                n185 = property on="IP Address_TSL1" class="Str"("DisabledEnum"=w281) -> ()  [unwired: 2 in, 2 out]
              }
            }
          }
          event "Communication_PCU": Value Change {
            n186 = event-data() -> ()  [unwired: 1 in, 6 out]
            n187 = case shown="\"rdopcu_gpib\", Default" "Communication_PCU" {
              frame "rdopcu_gpib", Default {
                w284 = T4."Disabled and Grayed Out" ("禁用")
                # "PCU Communcatior GPIB Checked"
                n188 = property on="txtpcu_ipadd" class="Str"("DisabledEnum"=w284) -> ()  [unwired: 2 in, 2 out]
                n189 = property on="txtpcu_gpibadd" class="DigNum (strict)"("DisabledEnum"=T4."Enabled" ("禁用")) -> ()  [unwired: 2 in, 2 out]
                n190 = property on="txtpcu_lanport" class="DigNum (strict)"("DisabledEnum"=w284) -> ()  [unwired: 2 in, 2 out]
                n191 = property on="cmbpcu_usbresource" class="Ring (strict)"("DisabledEnum"=w284) -> ()  [unwired: 2 in, 2 out]
              }
              frame "rdopcu_usb" {
                w287 = T4."Disabled and Grayed Out" ("禁用")
                # "PCU Communicator USB checked"
                n192 = property on="txtpcu_ipadd" class="Str"("DisabledEnum"=w287) -> ()  [unwired: 2 in, 2 out]
                n193 = property on="txtpcu_lanport" class="DigNum (strict)"("DisabledEnum"=w287) -> ()  [unwired: 2 in, 2 out]
                n194 = property on="txtpcu_gpibadd" class="DigNum (strict)"("DisabledEnum"=w287) -> ()  [unwired: 2 in, 2 out]
                n195 = property on="cmbpcu_usbresource" class="Ring (strict)"("DisabledEnum"=T4."Enabled" ("禁用")) -> ()  [unwired: 2 in, 2 out]
              }
              frame "rdopcu_lan" {
                w289 = T4."Disabled and Grayed Out" ("禁用")
                w288 = T4."Enabled" ("禁用")
                # "PCU communcatior TCP/IP Checked"
                n196 = property on="cmbpcu_usbresource" class="Ring (strict)"("DisabledEnum"=w289) -> ()  [unwired: 2 in, 2 out]
                n197 = property on="txtpcu_gpibadd" class="DigNum (strict)"("DisabledEnum"=w289) -> ()  [unwired: 2 in, 2 out]
                n198 = property on="txtpcu_ipadd" class="Str"("DisabledEnum"=w288) -> ()  [unwired: 2 in, 2 out]
                n199 = property on="txtpcu_lanport" class="DigNum (strict)"("DisabledEnum"=w288) -> ()  [unwired: 2 in, 2 out]
              }
            }
          }
          event "chkmulti_dev": Value Change {
            n200 = event-data() -> ()  [unwired: 1 in, 1 out]
            n201 = local read "chkmulti_dev"() -> (w292:bool)
            n202 = case shown="True" w292 {
              frame False {
                w293 = T4."Disabled and Grayed Out" ("禁用")
                n203 = property on="LAN Port_MPM 2" class="DigNum (strict)"("DisabledEnum"=w293) -> ()  [unwired: 2 in, 2 out]
                n204 = property on="IP Address_MPM 2" class="Str"("DisabledEnum"=w293) -> ()  [unwired: 2 in, 2 out]
                n205 = property on="GPIB Address_MPM 2" class="DigNum (strict)"("DisabledEnum"=w293) -> ()  [unwired: 2 in, 2 out]
              }
              frame True {
                n206 = local read "Communication_MPM"() -> (w294:enum32{"rdiGPIB_MPM", "rdiLAN_MPM"})
                n207 = case shown="\"rdiGPIB_MPM\", Default" w294 {
                  frame "rdiLAN_MPM" {
                    w295 = T4."Enabled" ("禁用")
                    n208 = property on="LAN Port_MPM 2" class="DigNum (strict)"("DisabledEnum"=w295) -> ()  [unwired: 2 in, 2 out]
                    n209 = property on="IP Address_MPM 2" class="Str"("DisabledEnum"=w295) -> ()  [unwired: 2 in, 2 out]
                    n210 = property on="GPIB Address_MPM 2" class="DigNum (strict)"("DisabledEnum"=T4."Disabled and Grayed Out" ("禁用")) -> ()  [unwired: 2 in, 2 out]
                  }
                  frame "rdiGPIB_MPM", Default {
                    w297 = T4."Disabled and Grayed Out" ("禁用")
                    n211 = property on="GPIB Address_MPM 2" class="DigNum (strict)"("DisabledEnum"=T4."Enabled" ("禁用")) -> ()  [unwired: 2 in, 2 out]
                    n212 = property on="IP Address_MPM 2" class="Str"("DisabledEnum"=w297) -> ()  [unwired: 2 in, 2 out]
                    n213 = property on="LAN Port_MPM 2" class="DigNum (strict)"("DisabledEnum"=w297) -> ()  [unwired: 2 in, 2 out]
                  }
                }
              }
            }
          }
          event "Communication_MPM": Value Change {
            n214 = event-data() -> ()  [unwired: 1 in, 1 out]
            n215 = local read "Communication_MPM"() -> (w301:enum32{"rdiGPIB_MPM", "rdiLAN_MPM"})
            n216 = case shown="\"rdiGPIB_MPM\", Default" w301 {
              frame "rdiLAN_MPM" {
                n217 = local read "chkmulti_dev"() -> (w302:bool)
                n218 = case shown="True" w302 {
                  frame True {
                    w303 = T4."Disabled and Grayed Out" ("禁用")
                    w304 = T4."Enabled" ("禁用")
                    n219 = property on="IP Address_MPM" class="Str"("DisabledEnum"=w304) -> ()  [unwired: 2 in, 2 out]
                    n220 = property on="LAN Port_MPM" class="DigNum (strict)"("DisabledEnum"=w304) -> ()  [unwired: 2 in, 2 out]
                    n221 = property on="LAN Port_MPM 2" class="DigNum (strict)"("DisabledEnum"=w304) -> ()  [unwired: 2 in, 2 out]
                    n222 = property on="IP Address_MPM 2" class="Str"("DisabledEnum"=w304) -> ()  [unwired: 2 in, 2 out]
                    n223 = property on="GPIB Address_MPM 2" class="DigNum (strict)"("DisabledEnum"=w303) -> ()  [unwired: 2 in, 2 out]
                    n224 = property on="GPIB Address_MPM" class="DigNum (strict)"("DisabledEnum"=w303) -> ()  [unwired: 2 in, 2 out]
                  }
                  frame False {
                    w305 = T4."Disabled and Grayed Out" ("禁用")
                    w306 = T4."Disabled and Grayed Out" ("禁用")
                    w307 = T4."Enabled" ("禁用")
                    n225 = property on="IP Address_MPM" class="Str"("DisabledEnum"=w307) -> ()  [unwired: 2 in, 2 out]
                    n226 = property on="LAN Port_MPM" class="DigNum (strict)"("DisabledEnum"=w307) -> ()  [unwired: 2 in, 2 out]
                    n227 = property on="IP Address_MPM 2" class="Str"("DisabledEnum"=w305) -> ()  [unwired: 2 in, 2 out]
                    n228 = property on="LAN Port_MPM 2" class="DigNum (strict)"("DisabledEnum"=w305) -> ()  [unwired: 2 in, 2 out]
                    n229 = property on="GPIB Address_MPM 2" class="DigNum (strict)"("DisabledEnum"=w306) -> ()  [unwired: 2 in, 2 out]
                    n230 = property on="GPIB Address_MPM" class="DigNum (strict)"("DisabledEnum"=w306) -> ()  [unwired: 2 in, 2 out]
                  }
                }
              }
              frame "rdiGPIB_MPM", Default {
                n231 = local read "chkmulti_dev"() -> (w308:bool)
                n232 = case shown="False" w308 {
                  frame True {
                    w309 = T4."Enabled" ("禁用")
                    w310 = T4."Disabled and Grayed Out" ("禁用")
                    n233 = property on="GPIB Address_MPM" class="DigNum (strict)"("DisabledEnum"=w309) -> ()  [unwired: 2 in, 2 out]
                    n234 = property on="GPIB Address_MPM 2" class="DigNum (strict)"("DisabledEnum"=w309) -> ()  [unwired: 2 in, 2 out]
                    n235 = property on="IP Address_MPM" class="Str"("DisabledEnum"=w310) -> ()  [unwired: 2 in, 2 out]
                    n236 = property on="LAN Port_MPM" class="DigNum (strict)"("DisabledEnum"=w310) -> ()  [unwired: 2 in, 2 out]
                    n237 = property on="IP Address_MPM 2" class="Str"("DisabledEnum"=w310) -> ()  [unwired: 2 in, 2 out]
                    n238 = property on="LAN Port_MPM 2" class="DigNum (strict)"("DisabledEnum"=w310) -> ()  [unwired: 2 in, 2 out]
                  }
                  frame False {
                    w311 = T4."Disabled and Grayed Out" ("禁用")
                    n239 = property on="GPIB Address_MPM" class="DigNum (strict)"("DisabledEnum"=T4."Enabled" ("禁用")) -> ()  [unwired: 2 in, 2 out]
                    n240 = property on="GPIB Address_MPM 2" class="DigNum (strict)"("DisabledEnum"=w311) -> ()  [unwired: 2 in, 2 out]
                    n241 = property on="LAN Port_MPM" class="DigNum (strict)"("DisabledEnum"=w311) -> ()  [unwired: 2 in, 2 out]
                    n242 = property on="LAN Port_MPM 2" class="DigNum (strict)"("DisabledEnum"=w311) -> ()  [unwired: 2 in, 2 out]
                    n243 = property on="IP Address_MPM 2" class="Str"("DisabledEnum"=w311) -> ()  [unwired: 2 in, 2 out]
                    n244 = property on="IP Address_MPM" class="Str"("DisabledEnum"=w311) -> ()  [unwired: 2 in, 2 out]
                  }
                }
              }
            }
          }
          event Panel Close? {
            n245 = event-data() -> ()  [unwired: 1 in, 4 out]
            n246 = event-data("Discard?"=TRUE ("放弃？")) -> ()  [unwired: 1 in, 1 out]
            "Boolean" <- FALSE
          }
        }
      }
    }
  }
  "Address Cluster out" <- w2
  "PowerMonitorType" <- w1
  n247 = call <vilib>:"General Error Handler.vi"("error in (no error)"=w5) -> ("error out"=→"错误输出":errorcluster)  [unwired: 10 in, 4 out]
